vi "Minimos.vi"(0 "Datos_IN":dbl[][](array[numeric]), 5 "Error In":errorcluster) -> (14 "Min_Array":dbl[](array[numeric]), 19 "Error Out":errorcluster)   [LabVIEW 2013]
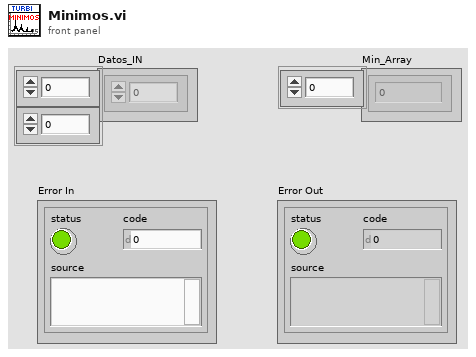
[diagram p1: front panel]
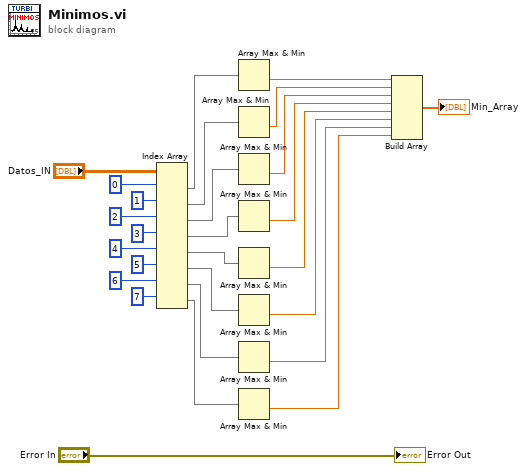
[diagram p0: block diagram]
diagram:
  n1 = Index Array(array="Datos_IN", index (row) #1=0 ("disabled index (col)"), index (row) #2=1 ("index (col)"), index (row) #3=2 ("index (col)"), index (row) #4=3 ("index (col)"), index (row) #5=4 ("index (col)"), index (row) #6=5 ("index (col)"), index (row) #7=6 ("index (col)"), index (row) #8=7 ("index (col)")) -> (element #1=w17:dbl[], element #2=w16:dbl[], element #3=w7:dbl[], element #4=w6:dbl[], element #5=w5:dbl[], element #6=w4:dbl[], element #7=w3:dbl[], element #8=w2:dbl[])  [unwired: 8 in]
  n2 = Array Max & Min(array=w17) -> (min value=w15:dbl)  [unwired: 3 out]
  n3 = Array Max & Min(array=w16) -> (min value=w14:dbl)  [unwired: 3 out]
  n4 = Array Max & Min(array=w7) -> (min value=w13:dbl)  [unwired: 3 out]
  n5 = Array Max & Min(array=w6) -> (min value=w12:dbl)  [unwired: 3 out]
  n6 = Array Max & Min(array=w5) -> (min value=w11:dbl)  [unwired: 3 out]
  n7 = Array Max & Min(array=w4) -> (min value=w10:dbl)  [unwired: 3 out]
  n8 = Array Max & Min(array=w3) -> (min value=w9:dbl)  [unwired: 3 out]
  n9 = Array Max & Min(array=w2) -> (min value=w8:dbl)  [unwired: 3 out]
  n10 = Build Array(w15, w14, w13, w12, w11, w10, w9, w8) -> (→"Min_Array":dbl[])
  "Error Out" <- "Error In"
